vi "Wait for Acquisition Complete.vi"(6 "Timeout (10000 ms)":i32=10000 min=1, 8 "error in (no error)":errorcluster, 11 "VISA resource name":refnum<visa-resource-name>) -> (0 "error out":errorcluster, 3 "VISA resource name out":refnum<visa-resource-name>)   [LabVIEW 2018, in "Yokogawa WT300 Series.lvlib"]
doc: "Detects whether the data aquisition is completed.\n\n<B>Note:</B> This VI does not check the instrument status. If you want to check the instrument status, call the Error Query VI at the conclusion of the sequence."
uses:
  Yokogawa WT300 Series.lvlib
panel:
  # "ms"
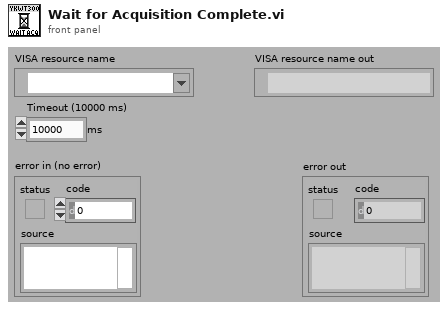
[diagram p1: front panel]
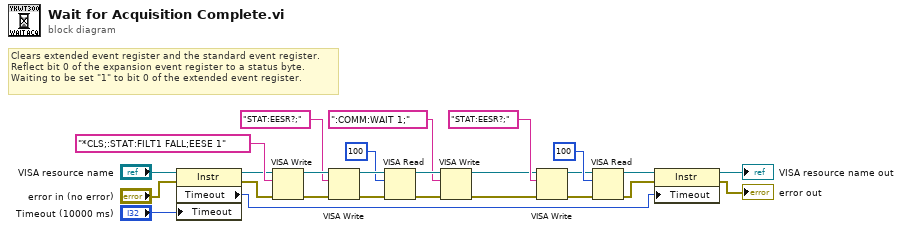
[diagram p0: block diagram]
diagram:
  # "Clears extended event register and the standard event register.\nReflect bit 0 of the expansion event register to a status byte.\nWaiting to be set \"1\" to bit 0 of the extended event register."
  n1 = property on="プロパティノード" class="Instr"(reference="VISA resource name", error in="error in (no error)", "Timeout"="Timeout (10000 ms)") -> (reference out=w13:refnum<visa-resource-name>, error out=w12:errorcluster, "Timeout"=w16:u32)
  n2 = VISA Write(VISA resource name=w13, write buffer="*CLS;:STAT:FILT1 FALL;EESE 1", error in (no error)=w12) -> (VISA resource name out=w24:refnum<visa-resource-name>, error out=w25:errorcluster)  [unwired: 1 out]
  n3 = VISA Write(VISA resource name=w24, write buffer="STAT:EESR?;", error in (no error)=w25) -> (VISA resource name out=w22:refnum<visa-resource-name>, error out=w23:errorcluster)  [unwired: 1 out]
  n4 = VISA Read(VISA resource name=w22, byte count=100, error in (no error)=w23) -> (VISA resource name out=w11:refnum<visa-resource-name>, error out=w10:errorcluster)  [unwired: 2 out]
  n5 = VISA Write ("VISA書き込み")(VISA resource name=w11, write buffer=":COMM:WAIT 1;", error in (no error)=w10) -> (VISA resource name out=w4:refnum<visa-resource-name>, error out=w3:errorcluster)  [unwired: 1 out]
  n6 = VISA Write(VISA resource name=w4, write buffer="STAT:EESR?;", error in (no error)=w3) -> (VISA resource name out=w7:refnum<visa-resource-name>, error out=w6:errorcluster)  [unwired: 1 out]
  n7 = VISA Read(VISA resource name=w7, byte count=100, error in (no error)=w6) -> (VISA resource name out=w2:refnum<visa-resource-name>, error out=w1:errorcluster)  [unwired: 2 out]
  n8 = property on="プロパティノード" class="Instr"(reference=w2, error in=w1, "Timeout"=w16) -> (reference out=→"VISA resource name out":refnum<visa-resource-name>, error out=→"error out":errorcluster)
